vi "ElevModeToDash.vi"(10 "Update?":bool, 11 "ElevModeIn":T1) -> (3 "ElevModeOut":T1)   [LabVIEW 2018]
uses:
  ElevModes.ctl
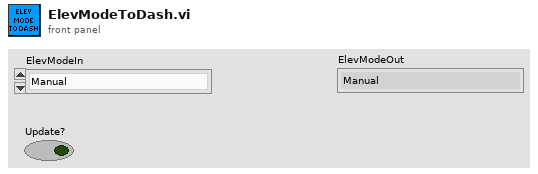
[diagram p1: front panel]
types:
  T1 = typedef "ElevModes.ctl" = enum16{"Manual", "Auto"}
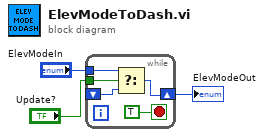
[diagram p0: block diagram]
diagram:
  n1 = while {
    tunnel: "Update?" -> [w8]
    tunnel: "ElevModeIn" -> [w7]
    shift-right: [w6] -> w1
    shift-left: _ -> [w5]
    stop <- TRUE stop-if-true
    n2 = Select(t=w7, s=w8, f=w5) -> (s? t:f=w6:T1)
  }
  "ElevModeOut" <- w1
